vi "Read_configuration_2ws.vi"(1 "configuration file path":path) -> (0 "output cluster":T1)   [LabVIEW 2015]
uses:
  <vilib>/LabVIEW Targets/FPGA/cRIO/shared/nicrio_ModuleControls/nicrio_cRIO-9234_DataRatesRing2.ctl
  <vilib>/Utility/config.llb/Read Key (Double).vi
  <vilib>/Utility/config.llb/Read Key (String).vi
  <vilib>/Utility/config.llb/Read Key (U32).vi
  <vilib>/Utility/config.llb/Read Key (Boolean).vi
  <vilib>/Utility/config.llb/NI_LVConfig.lvlib
panel:
  # "ID = 1"
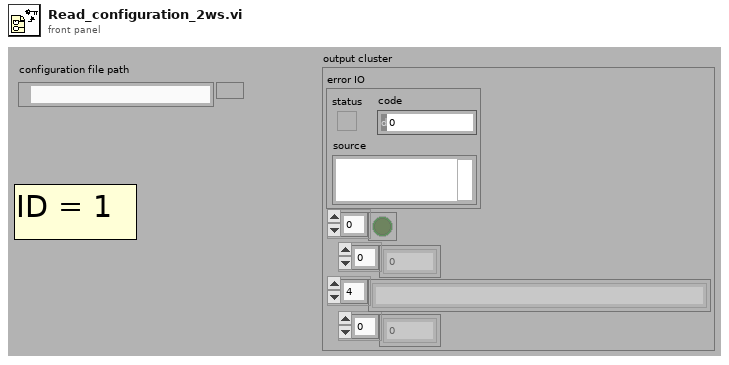
[diagram p1: front panel]
types:
  T1 = cluster{"error IO":errorcluster, bool[], u32[], string[], dbl[]}
  T2 = typedef "nicrio_cRIO-9234_DataRatesRing2.ctl" = u8
  T3 = typedef "NI_LVConfig.lvlib/Config Data RefNum.ctl" = refnum<k1>
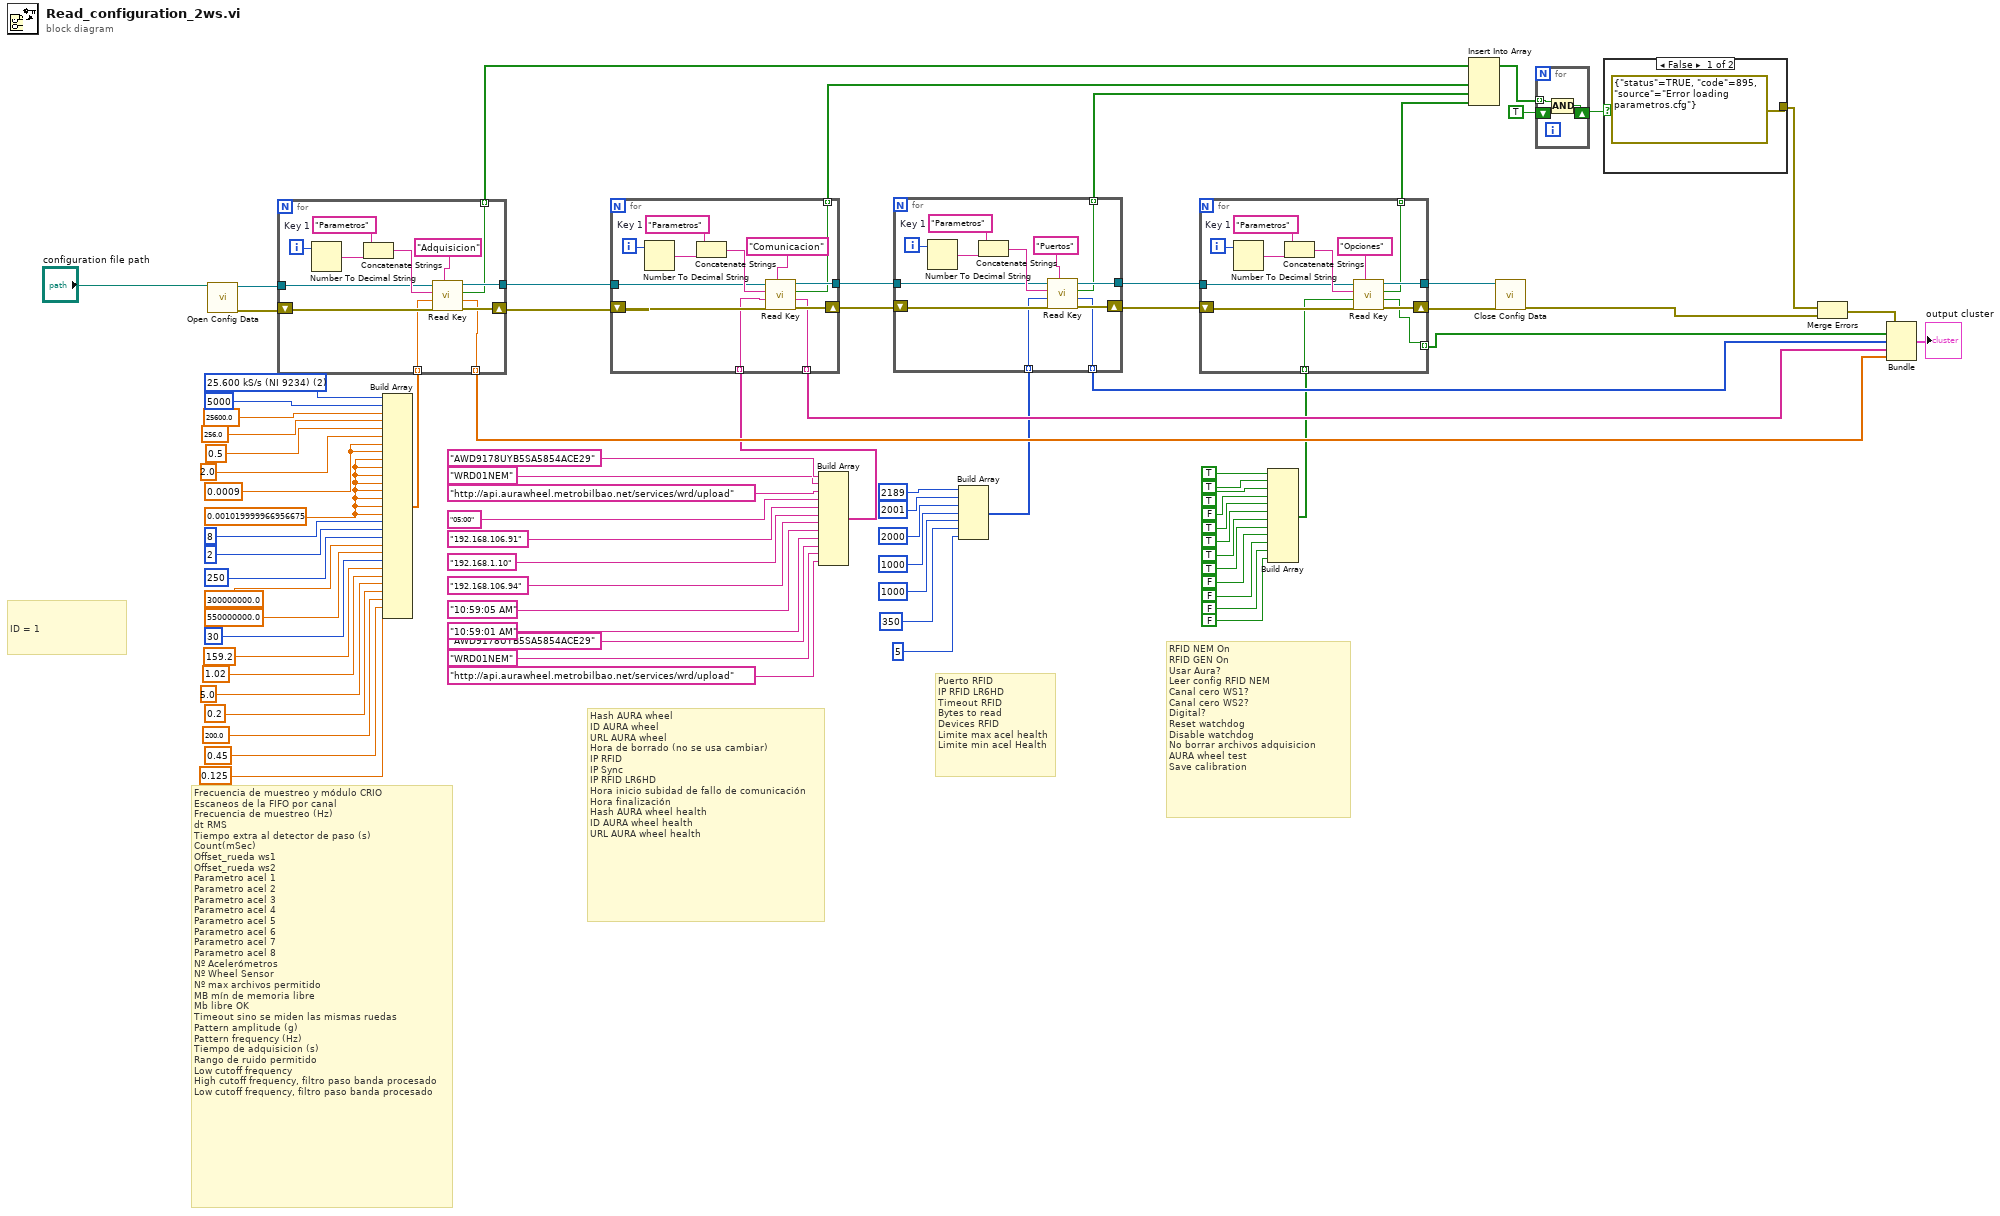
[diagram p0: block diagram]
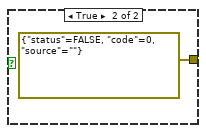
[diagram p2: hidden frame]
diagram:
  w37 = T2 2 items=["51.200 kS/s (NI 9234)"=1, "25.600 kS/s (NI 9234)"=2, "17.067 kS/s (NI 9234)"=3, "12.800 kS/s (NI 9234)"=4, "10.240 kS/s (NI 9234)"=5, "8.533 kS/s (NI 9234)"=6, "7.314 kS/s (NI 9234)"=7, "6.400 kS/s (NI 9234)"=8, "5.689 kS/s (NI 9234)"=9, "5.120 kS/s (NI 9234)"=10, "4.654 kS/s (NI 9234)"=11, "4.267 kS/s (NI 9234)"=12, "3.938 kS/s (NI 9234)"=13, "3.657 kS/s (NI 9234)"=14, "3.413 kS/s (NI 9234)"=15, "3.200 kS/s (NI 9234)"=16, "3.012 kS/s (NI 9234)"=17, "2.845 kS/s (NI 9234)"=18, "2.695 kS/s (NI 9234)"=19, "2.560 kS/s (NI 9234)"=20, "2.438 kS/s (NI 9234)"=21, "2.328 kS/s (NI 9234)"=22, "2.226 kS/s (NI 9234)"=23, "2.133 kS/s (NI 9234)"=24, "2.048 kS/s (NI 9234)"=25, "1.969 kS/s (NI 9234)"=26, "1.896 kS/s (NI 9234)"=27, "1.829 kS/s (NI 9234)"=28, "1.765 kS/s (NI 9234)"=29, "1.707 kS/s (NI 9234)"=30, "1.652 kS/s (NI 9234)"=31] ("Data Rate")
  w18 = 0.0009 ("element")
  w36 = sgl 0.00102
  # "RFID NEM On\nRFID GEN On\nUsar Aura?\nLeer config RFID NEM\nCanal cero WS1?\nCanal cero WS2?\nDigital?\nReset watchdog\nDisable watchdog\nNo borrar archivos adquisicion\nAURA wheel test\nSave calibration"
  # "Puerto RFID\nIP RFID LR6HD\nTimeout RFID\nBytes to read\nDevices RFID\nLimite max acel health\nLimite min acel Health"
  # "Hash AURA wheel\nID AURA wheel\nURL AURA wheel\nHora de borrado (no se usa cambiar)\nIP RFID\nIP Sync\nIP RFID LR6HD\nHora inicio subidad de fallo de comunicación\nHora finalización\nHash AURA wheel health\nID AURA wheel health\nURL AURA wheel health"
  # "Frecuencia de muestreo y módulo CRIO\nEscaneos de la FIFO por canal\nFrecuencia de muestreo (Hz)\ndt RMS\nTiempo extra al detector de paso (s)\nCount(mSec)\nOffset_rueda ws1\nOffset_rueda ws2\nParametro acel 1\nParametro acel 2\nParametro acel 3\nParametro acel 4\nParametro acel 5\nParametro acel 6\nParametro acel 7\nParametro acel 8\nNº Acelerómetros\nNº Wheel Sensor\nNº max archivos permitido\nMB mín de memoria libre\nMb libre OK\nTimeout sino se miden las mismas ruedas\nPattern amplitude (g)\nPattern frequency (Hz)\nTiempo de adquisicion (s)\nRango de ruido permitido\nLow cutoff frequency\nHigh cutoff frequency, filtro paso banda procesado\nLow cutoff frequency, filtro paso banda procesado"
  # "ID = 1"
  n1 = call <vilib>:"Open Config Data.vi"("configuration file path"="configuration file path") -> ("error out"=w54:errorcluster, "refnum"=w55:T3)  [unwired: 2 in, 7 out]
  n2 = Build Array(w37, 5000, 25600.0 ("element"), 256.0 ("element"), 0.5 ("element"), 2.0 ("element"), w18, w18, w36, w36, w36, w36, w36, w36, w36, w36, 8, 2, 250, 300000000.0, 550000000.0, 30, 159.2, 1.02, 5.0, 0.2, 200.0 ("element"), 0.45 ("element"), 0.125 ("element")) -> (w64:dbl[])
  n3 = for {
    tunnel: w55 -> [w89]
    shift-right: [w87] -> w50
    shift-left: w54 -> [w88]
    tunnel: [w86] -> w51
    tunnel: [w85] -> w82 mode=indexing
    tunnel: [w84] -> w53 mode=indexing
    tunnel: w64 -> [w83] mode=indexing
    i -> [w93]
    w91 = "Parametros"  # Key 1
    n4 = Number To Decimal String(number=w93) -> (decimal integer string=w92:string)  [unwired: 1 in]
    n5 = Concatenate Strings(w91, w92) -> (w90:string)
    n6 = call-poly <vilib>:"Read Key.vi"("section"="Adquisicion", "error in (no error)"=w88, "default value"=w83, "key"=w90, "refnum"=w89) -> ("error out"=w87:errorcluster, "value"=w85:dbl, "found?"=w84:bool, "refnum out"=w86:T3)  [unwired: 3 in]
  }
  n7 = Build Array("AWD9178UYB5SA5854ACE29" ("URL LOGIN"), "WRD01NEM" ("URL ENVÍO PARAM"), "http://api.aurawheel.metrobilbao.net/services/wrd/upload" ("URL LOGOUT"), "05:00", "192.168.106.91" ("element"), "192.168.1.10" ("Time Server\nIP Address"), "192.168.106.94" ("Time Server\nIP Address"), "10:59:05 AM" ("element"), "10:59:01 AM" ("element"), "AWD9178UYB5SA5854ACE29" ("URL LOGIN"), "WRD01NEM" ("URL ENVÍO PARAM"), "http://api.aurawheel.metrobilbao.net/services/wrd/upload" ("URL LOGOUT")) -> (w63:string[])
  n8 = for {
    tunnel: w51 -> [w101]
    shift-right: [w99] -> w73
    shift-left: w50 -> [w100]
    tunnel: [w98] -> w72
    tunnel: [w97] -> w81 mode=indexing
    tunnel: [w96] -> w49 mode=indexing
    tunnel: w63 -> [w95] mode=indexing
    i -> [w105]
    w103 = "Parametros"  # Key 1
    n9 = Number To Decimal String(number=w105) -> (decimal integer string=w104:string)  [unwired: 1 in]
    n10 = Concatenate Strings(w103, w104) -> (w102:string)
    n11 = call-poly <vilib>:"Read Key.vi"("section"="Comunicacion", "error in (no error)"=w100, "default value"=w95, "key"=w102, "refnum"=w101) -> ("error out"=w99:errorcluster, "value"=w97:string, "found?"=w96:bool, "refnum out"=w98:T3)  [unwired: 3 in]
  }
  n12 = Build Array(u16 2189 ("element"), u16 2001 ("element"), u16 2000 ("element"), u16 1000 ("element"), u16 1000 ("element"), u16 350 ("element"), u16 5 ("element")) -> (w62:u16[])
  n13 = for {
    tunnel: w72 -> [w113]
    shift-right: [w111] -> w75
    shift-left: w73 -> [w112]
    tunnel: [w110] -> w74
    tunnel: [w109] -> w80 mode=indexing
    tunnel: [w108] -> w48 mode=indexing
    tunnel: w62 -> [w107] mode=indexing
    i -> [w117]
    w115 = "Parametros"  # Key 1
    n14 = Number To Decimal String(number=w117) -> (decimal integer string=w116:string)  [unwired: 1 in]
    n15 = Concatenate Strings(w115, w116) -> (w114:string)
    n16 = call-poly <vilib>:"Read Key.vi"("section"="Puertos", "error in (no error)"=w112, "default value"=w107, "key"=w114, "refnum"=w113) -> ("error out"=w111:errorcluster, "value"=w109:u32, "found?"=w108:bool, "refnum out"=w110:T3)  [unwired: 3 in]
  }
  n17 = Build Array(TRUE, TRUE, TRUE, FALSE ("element"), TRUE ("element"), TRUE ("element"), TRUE ("element"), TRUE ("element"), FALSE ("element"), FALSE ("element"), FALSE ("element"), FALSE ("element")) -> (w59:bool[])
  n18 = for {
    tunnel: w74 -> [w125]
    shift-right: [w123] -> w76
    shift-left: w75 -> [w124]
    tunnel: [w122] -> w77
    tunnel: [w121] -> w79 mode=indexing
    tunnel: [w120] -> w47 mode=indexing
    tunnel: w59 -> [w119] mode=indexing
    i -> [w129]
    w127 = "Parametros"  # Key 1
    n19 = Number To Decimal String(number=w129) -> (decimal integer string=w128:string)  [unwired: 1 in]
    n20 = Concatenate Strings(w127, w128) -> (w126:string)
    n21 = call-poly <vilib>:"Read Key.vi"("section"="Opciones", "error in (no error)"=w124, "default value"=w119, "key"=w126, "refnum"=w125) -> ("error out"=w123:errorcluster, "value"=w121:bool, "found?"=w120:bool, "refnum out"=w122:T3)  [unwired: 3 in]
  }
  n22 = Insert Into Array(array=w53, new element #1=w49, new element #2=w48, new element #3=w47) -> (w56:bool[])  [unwired: 1 in]
  n23 = call <vilib>:"Close Config Data.vi"("error in (no error)"=w76, "refnum"=w77) -> ("error out"=w70:errorcluster)  [unwired: 8 in, 1 out]
  n24 = for {
    shift-right: [w132] -> w57
    shift-left: TRUE -> [w133]
    tunnel: w56 -> [w131] mode=indexing
    n25 = Compound Arithmetic op=AND(w131, w133) -> (w132:bool)
  }
  n26 = case shown="False" w57 {
    tunnel: [errorcluster {"status"=TRUE, "code"=895, "source"="Error loading parametros.cfg"} ("error out") errorcluster {"status"=FALSE, "code"=0, "source"=""} ("error out")] -> w71
    frame False {
    }
    frame True {
    }
  }
  n27 = Merge Errors(w71, w70) -> (w69:errorcluster)
  n28 = Bundle("error IO"=w69, w79, w80, w81, w82) -> (→"output cluster":T1)  [unwired: 1 in]
